vi "Start Result Waveforms (First Call).vi"(8 "error in (no error)":errorcluster, 9 "Properties":T1, 10 "First Call?":bool, 11 "Result Wfm Session Ref":refnum<class "Single Waveform Write (DBL).lvclass">) -> (0 "error out":errorcluster)   [LabVIEW 2020, in "Waveform-Processing-Custom-Device Engine.lvlib"]
uses:
  Waveform-Processing-Custom-Device Engine.lvlib
  <vilib>/NI VeriStand/Custom Device Waveform API/Single Waveform Write (DBL)/Single Waveform Write (DBL).lvclass
  C:/Program Files (x86)/National Instruments/LabVIEW 2020/vi.lib/NI VeriStand/Custom Device Waveform API/Waveform Session.lvclass
  <vilib>/NI VeriStand/Custom Device Waveform API/Waveform properties.ctl
  <vilib>/NI VeriStand/Custom Device API/Waveform Data Reference.ctl
  <vilib>/NI VeriStand/Custom Device Waveform API/Waveform Session.lvclass/Waveform Session.ctl
  <vilib>/NI VeriStand/Custom Device Waveform API/Single Waveform Write (DBL)/Single Waveform Write (DBL).lvclass/Single Waveform Write (DBL).ctl
  <vilib>/NI VeriStand/Custom Device Waveform API/Internal Comm Classes/WPL Comm/WPL Comm.lvclass/WPL Comm.ctl
  <vilib>/NI VeriStand/Custom Device Waveform API/Single Waveform Write (DBL)/NI VeriStand - Start Single Waveform (DBL).vi
  <vilib>/NI VeriStand/Custom Device Waveform API/Internal Comm Classes/WPL Comm/WPL_start dbl waveform.vi
  <vilib>/NI VeriStand/Custom Device Waveform API/Read Sample offset DVR.vi
  <vilib>/NI VeriStand/Custom Device Waveform API/Check Opened.vi
  <vilib>/NI VeriStand/Custom Device Waveform API/Internal Comm Classes/WPL Comm/Set t0 on Variant.vi
  <vilib>/NI VeriStand/Custom Device Waveform API/Internal Comm Classes/WPL Comm/Send WPL Command.vi
  <vilib>/NI VeriStand/Custom Device Waveform API/Internal Comm Classes/WPL Comm/Convert Q Error to Shutdown Error.vi
  <vilib>/NI VeriStand/Custom Device Waveform API/Internal Comm Classes/WPL Comm/WPL Comm (1D DBL)/WPL Comm (1D DBL).lvclass
  C:/Program Files (x86)/National Instruments/LabVIEW 2020/vi.lib/NI VeriStand/Custom Device Waveform API/Internal Comm Classes/WPL Comm/WPL Comm.lvclass
  <vilib>/Utility/error.llb/Error Cluster From Error Code.vi
  <vilib>/NI VeriStand/Custom Device Waveform API/NI_VS Custom Device Waveform API.lvlib
  <vilib>/NI VeriStand/Custom Device API/Custom Device API.lvlib
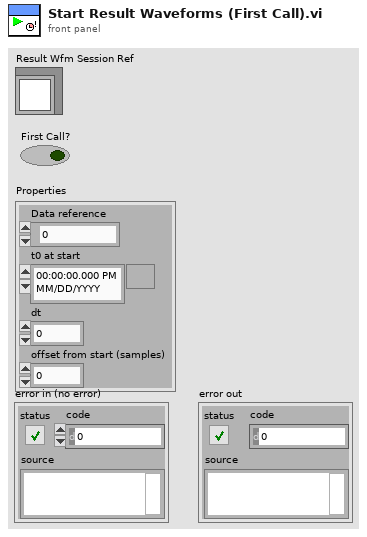
[diagram p1: front panel]
types:
  T1 = typedef "NI_VS Custom Device Waveform API.lvlib/Waveform properties.ctl" = cluster{"Data reference":T2, "t0 at start":timestamp, "dt":dbl, "offset from start (samples)":u64}
  T2 = typedef "Custom Device API.lvlib/Waveform Data Reference.ctl" = i32
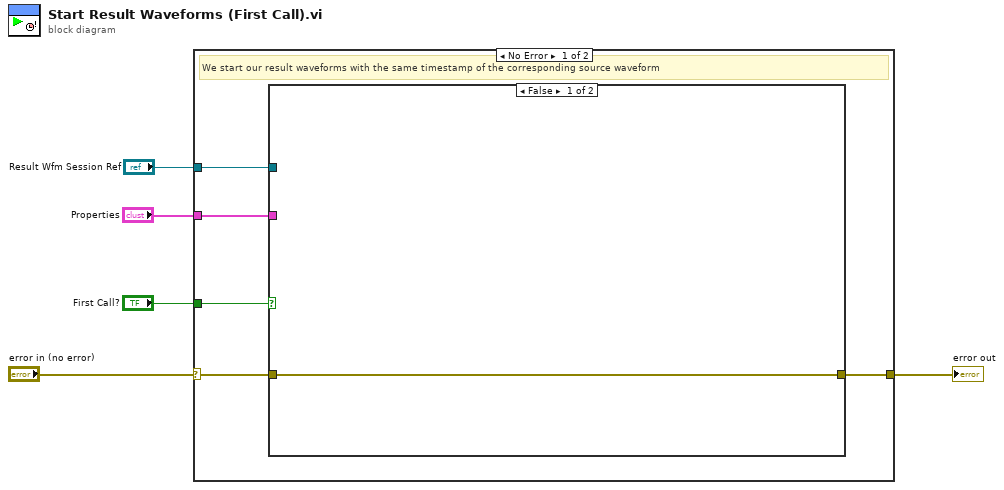
[diagram p0: block diagram]
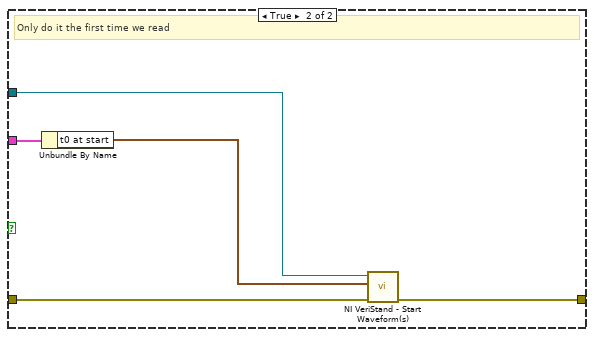
[diagram p2: hidden frame]
diagram:
  n1 = case shown="No Error" "error in (no error)" {
    selector: "error in (no error)" -> [w7 w17]
    tunnel: [w6 w17] -> w4
    tunnel: "Result Wfm Session Ref" -> [w9 _]
    tunnel: "Properties" -> [w8 _]
    tunnel: "First Call?" -> [w10 _]
    frame No Error {
      # "We start our result waveforms with the same timestamp of the corresponding source waveform"
      n2 = case shown="False" w10 {
        tunnel: w9 -> [_ w14]
        tunnel: w8 -> [_ w13]
        tunnel: w7 -> [w11 w16]
        tunnel: [w11 w15] -> w6
        frame False {
        }
        frame True {
          # "Only do it the first time we read"
          n3 = Unbundle By Name(w13) -> ("t0 at start"=w12:timestamp)
          n4 = call-poly <vilib>:"NI VeriStand - Start Waveform(s).vi"("error in (no error)"=w16, "t0"=w12, "Single Waveform Write Session (DBL) in"=w14) -> ("error out"=w15:errorcluster)  [unwired: 7 in, 1 out]
        }
      }
    }
    frame Error {
    }
  }
  "error out" <- w4
